vi "Modbus Settings from INI.vi"(8 "error in":errorcluster, 11 "Config Refnum in":T3) -> (0 "error out":errorcluster, 3 "Config Refnum out":T3, 4 "Modbus Configuration":T1)   [LabVIEW 2018, in "AE75TX Actor.lvlib" / "AE75TX.lvclass"]
uses:
  AE75TX.lvclass
  <vilib>/Utility/config.llb/Config Data RefNum.ctl
  Controls/Modbus Configuration Cluster.ctl
  <vilib>/ORNL/CSEISMIC DDS/CSEISMIC DDS Base/Data Types/Controls/DeviceID.ctl
  <vilib>/Utility/config.llb/Read Key (String).vi
  <vilib>/Utility/config.llb/Read Key (U32).vi
  <vilib>/Utility/config.llb/NI_LVConfig.lvlib
  <vilib>/ORNL/CSEISMIC DDS/CSEISMIC DDS Base/CSEISMIC DDS.lvclass
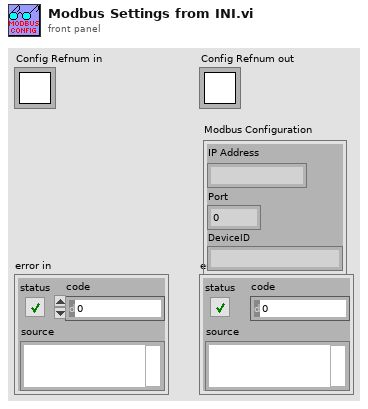
[diagram p1: front panel]
types:
  T1 = typedef "AE75TX Actor.lvlib/AE75TX.lvclass/Modbus Configuration Cluster.ctl" = cluster{"IP Address":string, "Port":u16, "DeviceID":T2}
  T2 = typedef "CSEISMIC DDS.lvlib/CSEISMIC DDS.lvclass/DeviceID.ctl" = string
  T3 = typedef "NI_LVConfig.lvlib/Config Data RefNum.ctl" = refnum<k1>
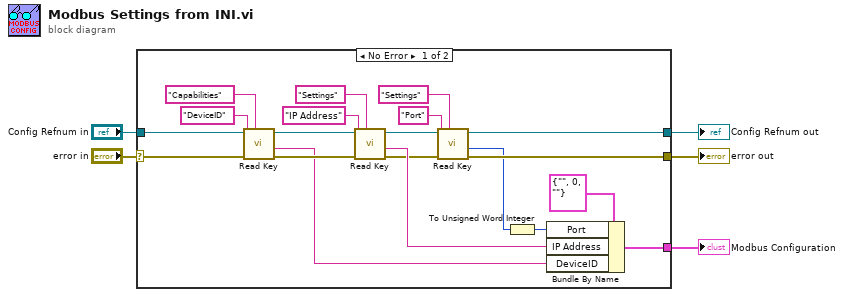
[diagram p0: block diagram]
diagram:
  n1 = case shown="No Error" "error in" {
    selector: "error in" -> [w7 w27]
    tunnel: [w16 w27] -> w5
    tunnel: [w17 w26] -> w4
    tunnel: [w25 _] -> w1
    tunnel: "Config Refnum in" -> [w8 w26]
    frame No Error {
      n2 = call-poly <vilib>:"Read Key.vi"("section"="Capabilities", "error in (no error)"=w7, "key"="DeviceID", "refnum"=w8) -> ("error out"=w10:errorcluster, "value"=w6:string, "refnum out"=w9:T3)  [unwired: 4 in, 1 out]
      n3 = call-poly <vilib>:"Read Key.vi"("section"="Settings", "error in (no error)"=w10, "key"="IP Address", "refnum"=w9) -> ("error out"=w19:errorcluster, "value"=w22:string, "refnum out"=w18:T3)  [unwired: 4 in, 1 out]
      n4 = call-poly <vilib>:"Read Key.vi"("section"="Settings", "error in (no error)"=w19, "key"="Port", "refnum"=w18) -> ("error out"=w16:errorcluster, "value"=w15:u32, "refnum out"=w17:T3)  [unwired: 4 in, 1 out]
      n5 = To Unsigned Word Integer(number=w15) -> (unsigned 16bit integer=w13:u16)
      n6 = Bundle By Name(cluster=T1 {"IP Address"="", "Port"=0, "DeviceID"=""} ("Modbus Configuration"), "Port"=w13, "IP Address"=w22, "DeviceID"=w6) -> (w25:T1)
    }
    frame Error {
    }
  }
  "error out" <- w5
  "Config Refnum out" <- w4
  "Modbus Configuration" <- w1
